vi "finishUp.vi"(8 "error in (no error)":errorcluster, 11 "ScanCreator in":refnum<class "ScanCreator.lvclass">) -> (0 "error out":errorcluster, 3 "ScanCreator out":refnum<class "ScanCreator.lvclass">)   [LabVIEW 2011, in "Views.lvlib" / "ScriptEditor.lvlib" / "ScanCreator.lvclass"]
uses:
  ScanCreator.lvclass
  ScanCreator.lvclass/ScanCreator.ctl
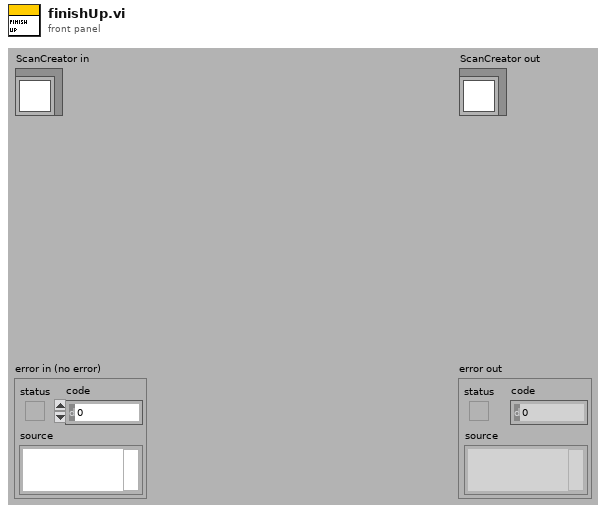
[diagram p1: front panel]
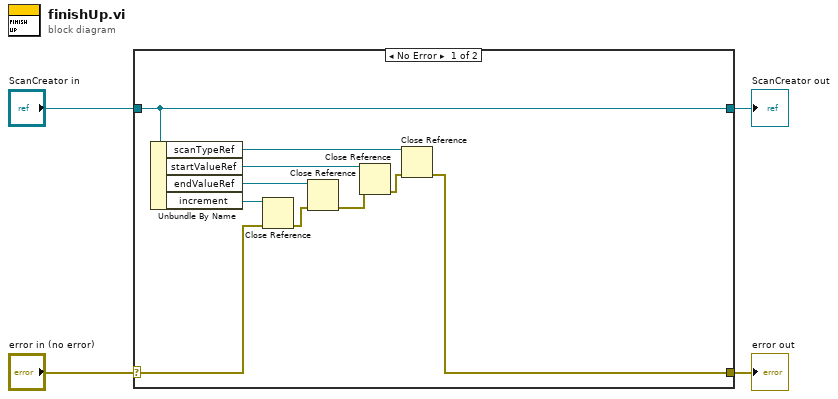
[diagram p0: block diagram]
diagram:
  n1 = case shown="No Error" "error in (no error)" {
    selector: "error in (no error)" -> [w6 w16]
    tunnel: [w5 w16] -> w3
    tunnel: [w14 w15] -> w1
    tunnel: "ScanCreator in" -> [w14 w15]
    frame No Error {
      n2 = Unbundle By Name(w14) -> ("scanTypeRef"=w10:refnum<vi>, "startValueRef"=w11:refnum<vi>, "endValueRef"=w12:refnum<vi>, "increment"=w13:refnum<vi>)
      n3 = Close Reference(reference=w13, error in (no error)=w6) -> (error out=w7:errorcluster)
      n4 = Close Reference(reference=w12, error in (no error)=w7) -> (error out=w8:errorcluster)
      n5 = Close Reference(reference=w11, error in (no error)=w8) -> (error out=w9:errorcluster)
      n6 = Close Reference(reference=w10, error in (no error)=w9) -> (error out=w5:errorcluster)
    }
    frame Error {
    }
  }
  "error out" <- w3
  "ScanCreator out" <- w1
